vi "rad_Add Target By IP Dialog.vi"() -> (2 "Canceled?":bool, 3 "IP Address":string)   [LabVIEW 2014]
panel:
  in  "Cancel":bool
  in  "View Target Info":bool
  in  "IP Address":string
  out "Target Information":string[][](table)
  in  "Add":bool
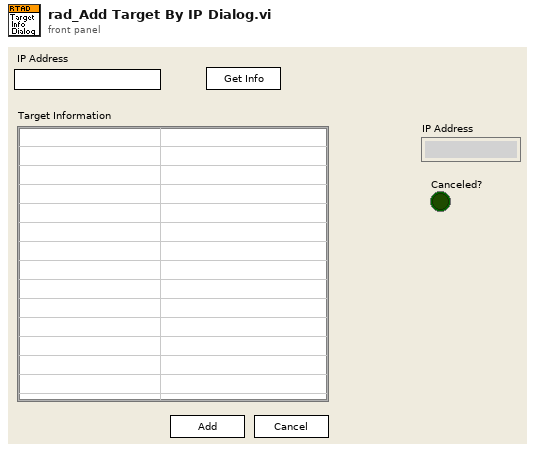
[diagram p1: front panel]
types:
  T1 = enum8{"Enabled", "Disabled", "Disabled and Grayed Out"}
  T2 = typedef "rad_Target Information.ctl" = cluster{"Hostname":string, "Serial number":string, "Product name":string, "Product code":i32, "System status":string, "Credential type":enum16{"None/Unlocked", "FTP Password", "NIAuth Credentials"}, "User added?":bool, "Primary NIC":T3}
  T3 = typedef "rad_Target Network Settings.ctl" = cluster{"MAC address":string, "IP Address Request Mode":i32, "IP address":string, "Subnet mask":string, "Gateway":string, "DNS server":string}
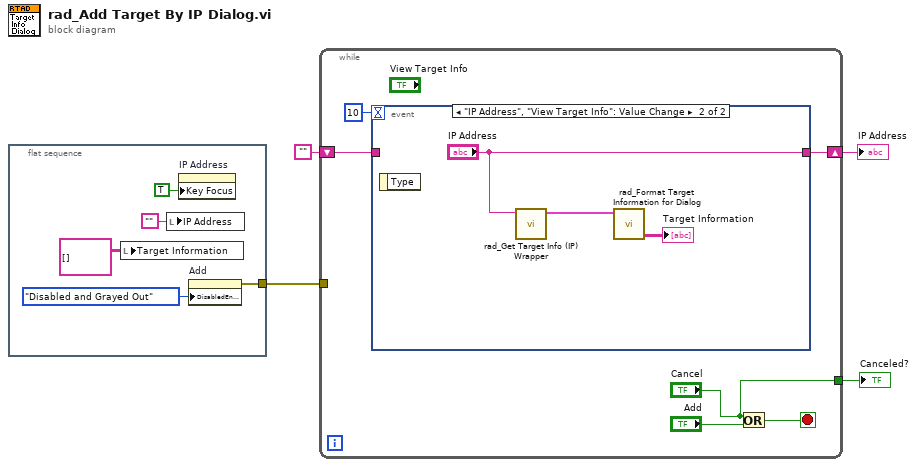
[diagram p0: block diagram]
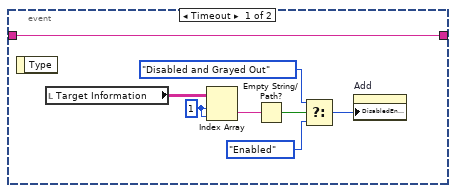
[diagram p2: hidden frame]
diagram:
  n1 = flat-sequence {
    tunnel: [w8] -> w3
    frame #0 {
      n2 = local write "Target Information"(string[][] [] ("Target Information")) -> ()
      n3 = local write "IP Address"("" ("IP Address")) -> ()
      n4 = property on="IP Address" class="Str"("Key Focus"=TRUE) -> ()  [unwired: 2 in, 2 out]
      n5 = property on="Add" class="Bool"("DisabledEnum"=T1."Disabled and Grayed Out" ("Disabled")) -> (error out=w8:errorcluster)  [unwired: 2 in, 1 out]
    }
  }
  n6 = while {
    tunnel: ["Cancel"] -> w4
    tunnel: w3 -> [_]
    shift-right: [w11] -> w2
    shift-left: "" ("IP Address") -> [w10]
    stop <- w14 stop-if-true
    n7 = event shown="[1] \"IP Address\", \"View Target Info\": Value Change" {
      selector: _ -> [_ _]
      dyn-events: _ -> [_ _]
      timeout: 10 -> [_ _]
      tunnel: [w17 "IP Address"] -> w11
      tunnel: w10 -> [w17 _]
      event Timeout {
        w22 = 1 ("index (row)")
        n8 = event-data() -> ()  [unwired: 1 in, 1 out]
        n9 = local read "Target Information"() -> (w23:string[][])
        n10 = Index Array(array=w23, index (row)=w22, index (col)=w22) -> (element=w16:string)
        n11 = Empty String/Path?(string/path=w16) -> (empty?=w21:bool)
        n12 = Select(t=T1."Disabled and Grayed Out" ("Disabled"), s=w21, f=T1."Enabled" ("Disabled")) -> (s? t:f=w18:T1)
        n13 = property on="Add" class="Bool"("DisabledEnum"=w18) -> ()  [unwired: 2 in, 2 out]
      }
      event "IP Address", "View Target Info": Value Change {
        n14 = event-data() -> ()  [unwired: 1 in, 1 out]
        n15 = call "rad_Get Target Info (IP) Wrapper.vi"("target address"="IP Address") -> ("Target settings"=w25:T2)  [unwired: 9 in, 1 out]
        n16 = call "rad_Format Target Information for Dialog.vi"("target settings in"=w25) -> ("Target Information"=→"Target Information":string[][])  [unwired: 9 in, 1 out]
      }
    }
    n17 = Or(x="Cancel", y="Add") -> (x .or. y?=w14:bool)
  }
  "Canceled?" <- w4
  "IP Address" <- w2
